vi "AquisicaoPeloSuper_adq.vi"() -> ()   [LabVIEW 2019]
panel:
  in  "PARAR":bool
  in  "Tempo":dbl
  out "reference_ADQ":refnum<vi>
  in  "error in (no error)":errorcluster
  in  "Frequencia":dbl
  out "Array":dbl[][](array[numeric])
  out "L reference":refnum<vi>
  out "C reference":refnum<vi>
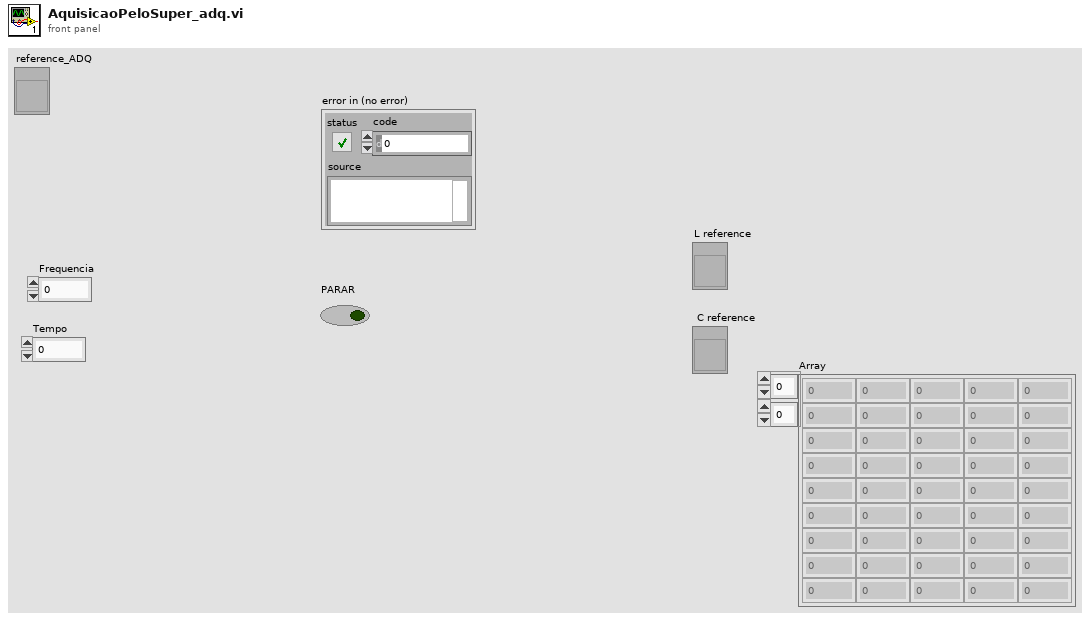
[diagram p1: front panel]
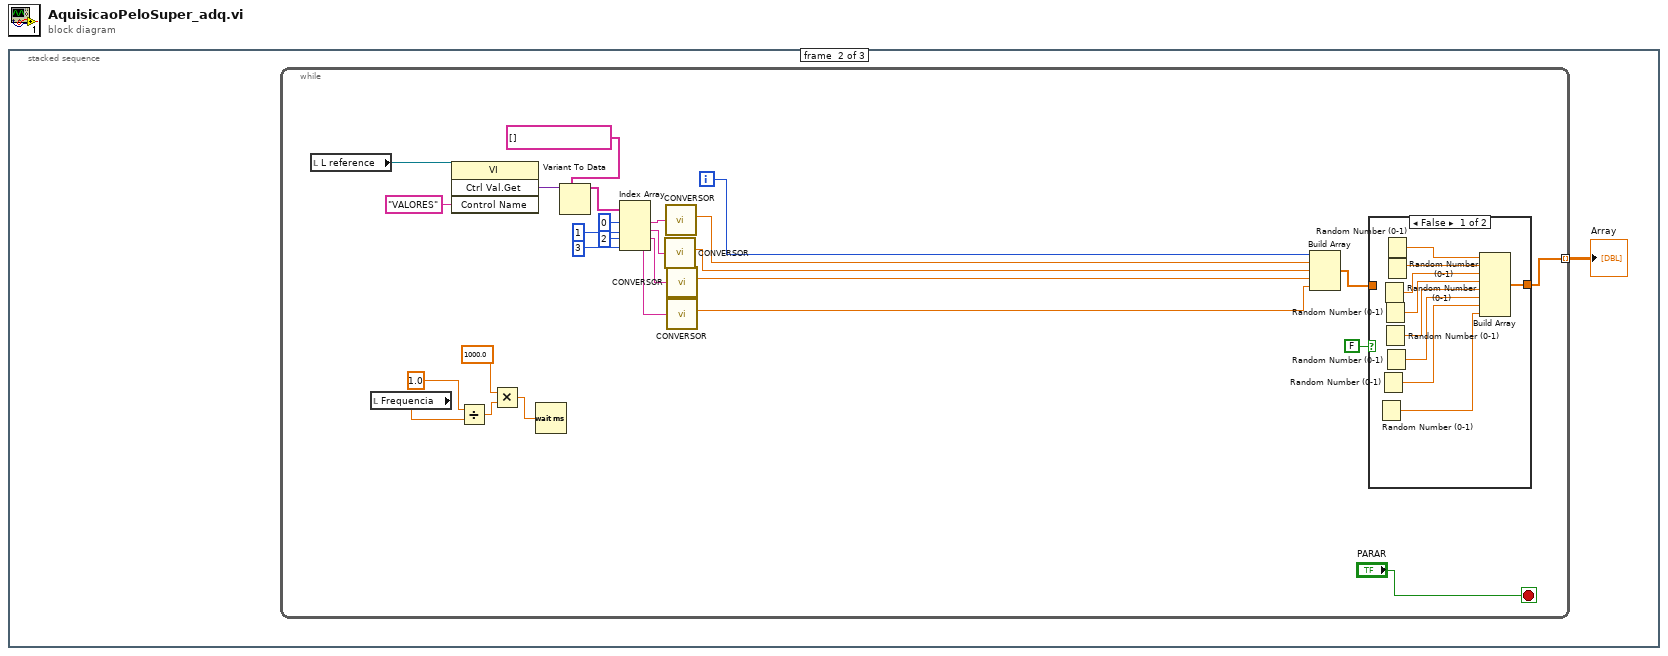
[diagram p0: block diagram]
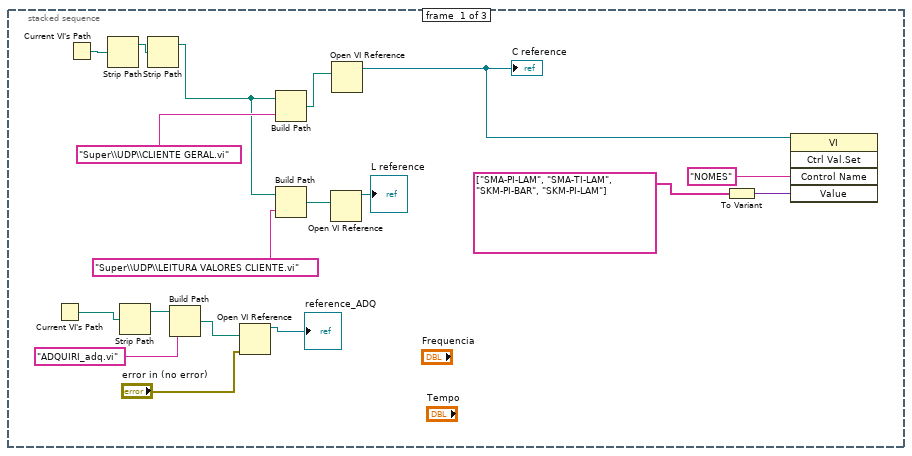
[diagram p2: hidden frame]
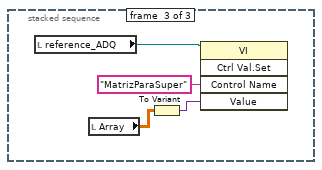
[diagram p4: hidden frame]
diagram:
  n1 = stacked-sequence {
    frame #0 {
      n2 = Current VI's Path() -> (path=w6:path)
      n3 = Current VI's Path() -> (path=w18:path)
      n4 = Strip Path(path=w18) -> (stripped path=w17:path)  [unwired: 1 out]
      n5 = Strip Path(path=w6) -> (stripped path=w4:path)  [unwired: 1 out]
      n6 = Strip Path(path=w17) -> (stripped path=w7:path)  [unwired: 1 out]
      n7 = Build Path(base path=w4, name or relative path="ADQUIRI_adq.vi") -> (appended path=w3:path)
      n8 = Open VI Reference(vi path=w3, error in (no error)="error in (no error)") -> (vi reference=→"reference_ADQ":refnum<vi>)  [unwired: 4 in, 1 out]
      n9 = Build Path(base path=w7, name or relative path="Super\\UDP\\CLIENTE GERAL.vi") -> (appended path=w15:path)
      n10 = Build Path(base path=w7, name or relative path="Super\\UDP\\LEITURA VALORES CLIENTE.vi") -> (appended path=w13:path)
      n11 = Open VI Reference(vi path=w13) -> (vi reference=→"L reference":refnum<vi>)  [unwired: 5 in, 1 out]
      n12 = Open VI Reference(vi path=w15) -> (vi reference=w8:refnum<vi>)  [unwired: 5 in, 1 out]
      "C reference" <- w8
      n13 = To Variant(anything=string[] ["SMA-PI-LAM", "SMA-TI-LAM", "SKM-PI-BAR", "SKM-PI-LAM"] ("NOMES")) -> (Variant=w10:variant)
      n14 = invoke class="VI" method="Ctrl Val.Set"(reference=w8, "Control Name"="NOMES", "Value"=w10) -> ()  [unwired: 2 in, 5 out]
    }
    frame #1 {
      n15 = while {
        tunnel: [w32] -> w19 mode=indexing
        i -> [w21]
        stop <- "PARAR" stop-if-true
        n16 = local read "L reference"() -> (w46:refnum<vi>)
        n17 = local read "Frequencia"() -> (w25:dbl)
        n18 = invoke class="VI" method="Ctrl Val.Get"(reference=w46, "Control Name"="VALORES") -> ("Get Control Value Variant"=w34:variant)  [unwired: 2 in, 3 out]
        n19 = Divide(x=1.0, y=w25) -> (x/y=w23:dbl)
        n20 = Multiply(x=1000.0, y=w23) -> (x*y=w22:dbl)
        n21 = Wait (ms)(milliseconds to wait=w22) -> ()  [unwired: 1 out]
        n22 = Variant To Data(type=string[] [] ("Array"), Variant=w34) -> (data=w43:string[])  [unwired: 1 in, 1 out]
        n23 = Index Array(array=w43, index #1=0 ("index"), index #2=1 ("index"), index #3=2 ("index"), index #4=3 ("index")) -> (element #1=w42:string, element #2=w40:string, element #3=w39:string, element #4=w38:string)
        n24 = call "CONVERSOR.vi"("String"=w40) -> ("float"=w29:dbl)  [unwired: 6 in, 3 out]
        n25 = call "CONVERSOR.vi"("String"=w42) -> ("float"=w30:dbl)  [unwired: 6 in, 3 out]
        n26 = call "CONVERSOR.vi"("String"=w39) -> ("float"=w28:dbl)  [unwired: 6 in, 3 out]
        n27 = call "CONVERSOR.vi"("String"=w38) -> ("float"=w27:dbl)  [unwired: 6 in, 3 out]
        n28 = Build Array(w21, w30, w29, w28, w27) -> (w33:dbl[])
        n29 = case shown="False" FALSE {
          tunnel: [w54 w56] -> w32
          tunnel: w33 -> [_ w56]
          frame False {
            n30 = Random Number (0-1)() -> (number: 0 to 1=w47:dbl)
            n31 = Random Number (0-1)() -> (number: 0 to 1=w48:dbl)
            n32 = Random Number (0-1)() -> (number: 0 to 1=w52:dbl)
            n33 = Random Number (0-1)() -> (number: 0 to 1=w51:dbl)
            n34 = Random Number (0-1)() -> (number: 0 to 1=w50:dbl)
            n35 = Random Number (0-1)() -> (number: 0 to 1=w49:dbl)
            n36 = Random Number (0-1)() -> (number: 0 to 1=w55:dbl)
            n37 = Random Number (0-1)() -> (number: 0 to 1=w53:dbl)
            n38 = Build Array(w55, w53, w52, w51, w50, w49, w48, w47) -> (w54:dbl[])
          }
          frame True {
          }
        }
      }
      "Array" <- w19
    }
    frame #2 {
      n39 = local read "reference_ADQ"() -> (w60:refnum<vi>)
      n40 = local read "Array"() -> (w58:dbl[][])
      n41 = To Variant(anything=w58) -> (Variant=w57:variant)
      n42 = invoke class="VI" method="Ctrl Val.Set"(reference=w60, "Control Name"="MatrizParaSuper", "Value"=w57) -> ()  [unwired: 2 in, 5 out]
    }
  }
